vi "Do.vi"(8 "error in (no error)":errorcluster, 10 "Actor in":refnum<class "Actor.lvclass">, 11 "Set Output Value Msg":refnum<class "Set Output Value Msg.lvclass">) -> (0 "error out":errorcluster, 2 "Actor out":refnum<class "Actor.lvclass">)   [LabVIEW 2020, in "BNT_ULx.lvlib" / "Set Output Value Msg.lvclass"]
doc: "This VI delivers the message to the actor by calling the appropriate method(s) on the actor."
uses:
  Set Output Value Msg.lvclass
  <vilib>/ActorFramework/Actor/Actor.lvclass
  C:/User/Brand/LVP/CSPP/CSPP-Template/Packages/CSPP_Core/Messages/CSPP_PVUpdate Msg/CSPP_PVUpdate Msg.lvclass
  BNT_ULx-MCSV/BNT_ULx-MCSV.lvclass
  C:/Program Files (x86)/National Instruments/LabVIEW 2020/vi.lib/ActorFramework/Actor/Actor.lvclass
  CSPP_Core/Messages/CSPP_PVUpdate Msg/CSPP_PVUpdate Msg.lvclass/CSPP_PVUpdate Msg.ctl
  CSPP_Core/Classes/CSPP_ProcessVariables/ProcessVariable/PV.lvclass/PV.ctl
  Set Output Value Msg.lvclass/Set Output Value Msg.ctl
  CSPP_Core/Classes/CSPP_ProcessVariables/ProcessVariable/PV.lvclass
  <vilib>/regexp/Match Regular Expression.xnode
  CSPP_Core/Messages/CSPP_PVUpdate Msg/CSPP_PVUpdate Msg.lvclass
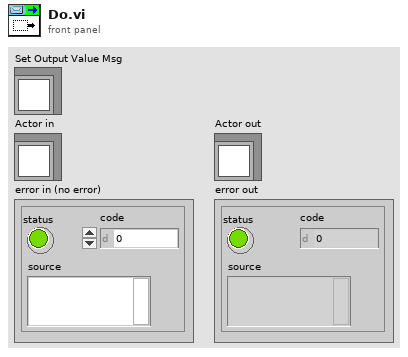
[diagram p1: front panel]
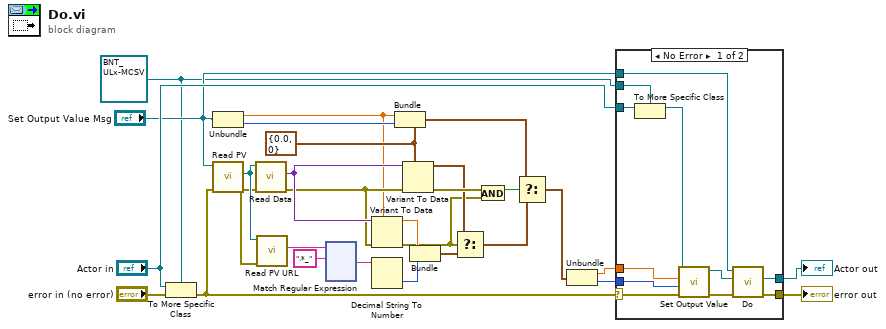
[diagram p0: block diagram]
diagram:
  w1 = refnum<class "BNT_ULx-MCSV.lvclass"> refnum ("BNT_ULx.lvlib:BNT_ULx-MCSV.lvclass")
  w21 = cluster{"Enable Channel":dbl, "Channel":i32} {"Enable Channel"=0.0, "Channel"=0} ("Type")
  n1 = To More Specific Class(target class=w1, reference="Actor in", error in="error in (no error)") -> (error out=w3:errorcluster)  [unwired: 1 out]
  n2 = Unbundle ("Pre-Unbundler")("Set Output Value Msg") -> (w10:dbl, w20:i32)
  n3 = call "Read PV.vi"("error in (no error)"=w3, "CS++PVUpdate Msg in"="Set Output Value Msg") -> ("error out"=w13:errorcluster, "PV"=w14:refnum<class "PV.lvclass">)  [unwired: 7 in, 1 out]
  n4 = call "Read Data.vi"("error in (no error)"=w13, "PV in"=w14) -> ("error out"=w11:errorcluster, "Data"=w12:variant)  [unwired: 7 in, 1 out]
  n5 = call "Read PV URL.vi"("error in (no error)"=w13, "PV in"=w14) -> ("PV URL"=w19:string)  [unwired: 7 in, 2 out]
  n6 = xnode "Match Regular Expression"("input string"=w19, "regular expression"=".*_") -> ("after match"=w17:string)  [unwired: 4 in, 4 out]
  n7 = Variant To Data(error in=w11, type=w10, Variant=w12) -> (data=w9:dbl, error out=w5:errorcluster)
  n8 = Decimal String To Number(string=w17) -> (number=w16:i32)  [unwired: 2 in, 1 out]
  n9 = Bundle ("Pre-Bundler")(cluster=w21, "Enable Channel"=w10, "Channel"=w20) -> (w22:cluster{"Enable Channel":dbl, "Channel":i32})
  n10 = Variant To Data(error in=w11, type=w21, Variant=w12) -> (data=w8:cluster{"Enable Channel":dbl, "Channel":i32}, error out=w23:errorcluster)
  n11 = Bundle ("Pre-Bundler")("Value"=w9, w16) -> (w15:cluster{"Value":dbl, i32})  [unwired: 1 in]
  n12 = Select ("MainSelect")(t=w8, s=w5, f=w15) -> (s? t:f=w7:cluster{"Value":dbl, "Channel":i32})
  n13 = And(x=w23, y=w5) -> (x .and. y?=w6:bool)
  n14 = Select ("MainSelect")(t=w22, s=w6, f=w7) -> (s? t:f=w2:cluster{"Value":dbl, "Channel":i32})
  n15 = Unbundle ("Main-Unbundler")(w2) -> ("Value"=w25:dbl, "Channel"=w24:i32)
  n16 = case shown="No Error" w3 {
    selector: w3 -> [w31 w42]
    tunnel: [w37 w42] -> w28
    tunnel: [w38 w41] -> w27
    tunnel: "Actor in" -> [w40 w41]
    tunnel: w1 -> [w39 _]
    tunnel: "Set Output Value Msg" -> [w36 _]
    tunnel: w25 -> [w33 _]
    tunnel: w24 -> [w32 _]
    frame No Error {
      n17 = To More Specific Class ("To More Specific Class (internal)")(target class=w39, reference=w40) -> (specific class reference=w35:refnum<class "BNT_ULx-MCSV.lvclass">)  [unwired: 1 in, 1 out]
      n18 = call "Set Output Value.vi"("Error In"=w31, "Channel"=w32, "Value"=w33, "BNT_ULx-MCSV in"=w35) -> ("Error Out"=w30:errorcluster, "BNT_ULx-MCSV out"=w34:refnum<class "BNT_ULx-MCSV.lvclass">)  [unwired: 6 in]
      n19 = call-parent "Do.vi"("error in (no error)"=w30, "Actor in"=w34, "CS++PVUpdate Msg"=w36) -> ("error out"=w37:errorcluster, "Actor out"=w38:refnum<class "Actor.lvclass">)  [unwired: 7 in]
    }
    frame Error {
    }
  }
  "error out" <- w28
  "Actor out" <- w27
